vi "DrawCircle.vi"(1 "Color":u32(colorbox)=6618880, 2 "Circle_D":i32, 3 "CircleCenterPosition":cluster{"x":sgl, "y":sgl}, 4 "Img in":T1) -> (0 "Img out":T1)   [LabVIEW 2014]
uses:
  <vilib>/vision/Image Controls.llb/IMAQ Image.ctl
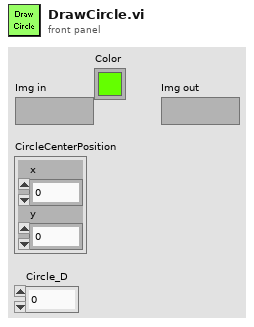
[diagram p1: front panel]
types:
  T1 = typedef "IMAQ Image.ctl" = refnum<image>
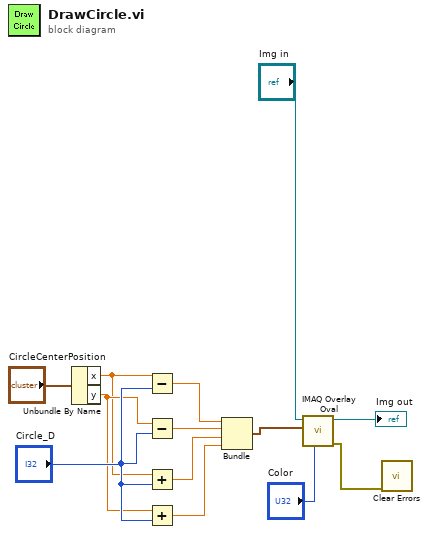
[diagram p0: block diagram]
diagram:
  n1 = Unbundle By Name("CircleCenterPosition") -> ("x"=w4:sgl, "y"=w5:sgl)
  n2 = Subtract(x=w4, y="Circle_D") -> (x-y=w7:sgl)
  n3 = Subtract(x=w5, y="Circle_D") -> (x-y=w8:sgl)
  n4 = Add(x=w4, y="Circle_D") -> (x+y=w9:sgl)
  n5 = Add(x=w5, y="Circle_D") -> (x+y=w10:sgl)
  n6 = Bundle(w7, w8, w9, w10) -> (w11:cluster{sgl, sgl, sgl, sgl})  [unwired: 1 in]
  n7 = call "IMAQ Overlay Oval"("Color"="Color", "Bounding Rectangle"=w11, "Image"="Img in") -> ("error out"=w1:errorcluster, "Image Out"=→"Img out":T1)  [unwired: 7 in]
  n8 = call <vilib>:"Clear Errors.vi"("error in (no error)"=w1) -> ()  [unwired: 5 in, 2 out]
